vi "Stats to Table.vi"(11 "Calculated Master WPC Stats":T1(array[cluster])) -> (3 "Calculated Stats Table":string[][](array[string]))   [LabVIEW 2021]
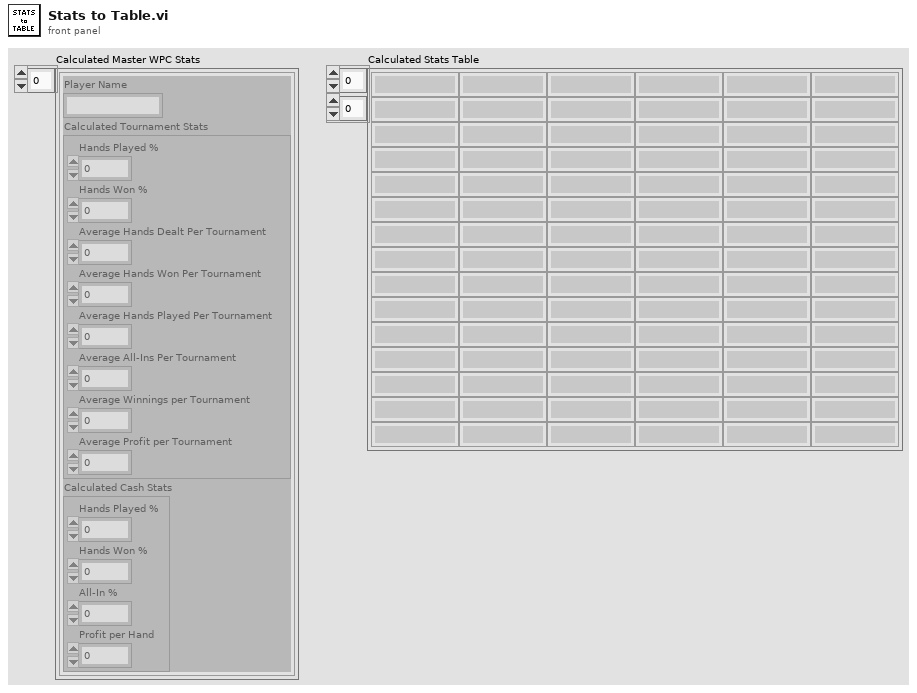
[diagram p1: front panel]
types:
  T1 = cluster{"Player Name":string, "Calculated Tournament Stats":cluster{"Hands Played %":dbl, "Hands Won %":dbl, "Average Hands Dealt Per Tournament":dbl, "Average Hands Won Per Tournament":dbl, "Average Hands Played Per Tournament":dbl, "Average All-Ins Per Tournament":dbl, "Average Winnings per Tournament":dbl, "Average Profit per Tournament":dbl}, "Calculated Cash Stats":cluster{"Hands Played %":dbl, "Hands Won %":dbl, "All-In %":dbl, "Profit per Hand":dbl}}[]
  T2 = cluster{"Hands Played %":dbl, "Hands Won %":dbl, "Average Hands Dealt Per Tournament":dbl, "Average Hands Won Per Tournament":dbl, "Average Hands Played Per Tournament":dbl, "Average All-Ins Per Tournament":dbl, "Average Winnings per Tournament":dbl, "Average Profit per Tournament":dbl}
  T3 = cluster{"Hands Played %":dbl, "Hands Won %":dbl, "All-In %":dbl, "Profit per Hand":dbl}
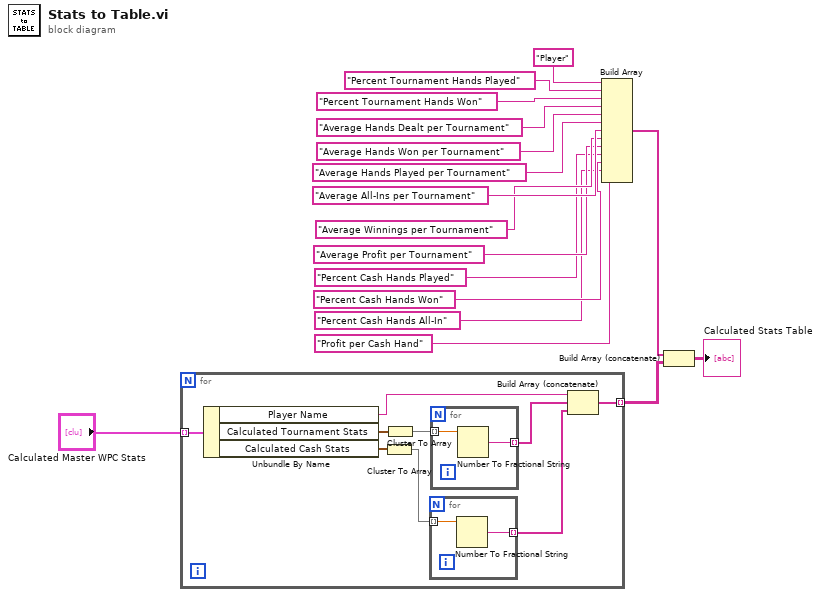
[diagram p0: block diagram]
diagram:
  n1 = for {
    tunnel: "Calculated Master WPC Stats" -> [w26] mode=indexing
    tunnel: [w18] -> w10 mode=indexing
    n2 = Unbundle By Name(w26) -> ("Player Name"=w21:string, "Calculated Tournament Stats"=w25:T2, "Calculated Cash Stats"=w24:T3)
    n3 = Cluster To Array(cluster=w24) -> (array=w22:dbl[])
    n4 = Cluster To Array(cluster=w25) -> (array=w23:dbl[])
    n5 = for {
      tunnel: w22 -> [w28] mode=indexing
      tunnel: [w27] -> w19 mode=indexing
      n6 = Number To Fractional String(number=w28) -> (F-format string=w27:string)  [unwired: 3 in]
    }
    n7 = for {
      tunnel: w23 -> [w30] mode=indexing
      tunnel: [w29] -> w20 mode=indexing
      n8 = Number To Fractional String(number=w30) -> (F-format string=w29:string)  [unwired: 3 in]
    }
    n9 = Build Array (concatenate)(w21, w20, w19) -> (w18:string[])
  }
  n10 = Build Array("Player", "Percent Tournament Hands Played", "Percent Tournament Hands Won", "Average Hands Dealt per Tournament", "Average Hands Won per Tournament", "Average Hands Played per Tournament", "Average All-Ins per Tournament", "Average Winnings per Tournament", "Average Profit per Tournament", "Percent Cash Hands Played", "Percent Cash Hands Won", "Percent Cash Hands All-In", "Profit per Cash Hand") -> (w11:string[])
  n11 = Build Array (concatenate)(w11, w10) -> (→"Calculated Stats Table":string[][])
